vi "AutomatedBeamWatch.vi"   [LabVIEW 2019]
uses:
  C:/Program Files/Spiricon/BeamWatch/BeamWatch.Automation.dll
  Program Files/Spiricon/BeamWatch/BeamWatch.Automation.dll
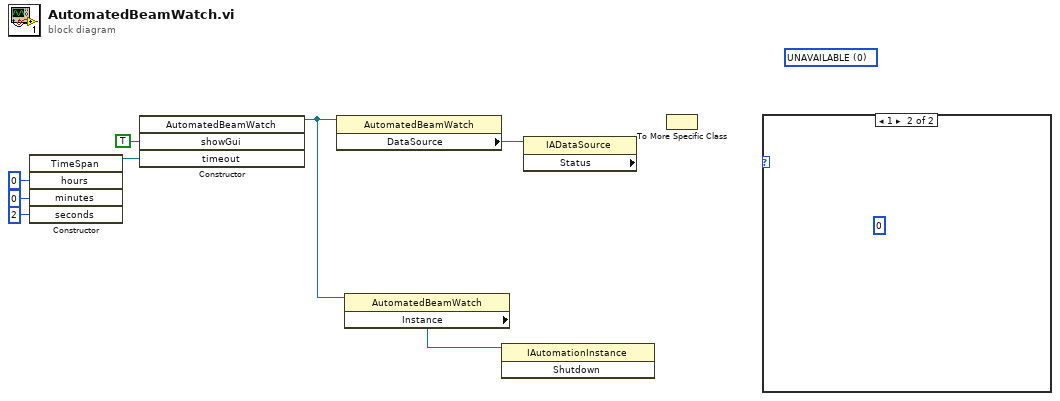
[diagram p0: block diagram]
diagram:
  (unwired) 0 items=["UNAVAILABLE", "RUNNING", "PAUSED"] ("Status")
  n1 = constructor class="TimeSpan"("hours"=0, "minutes"=0, "seconds"=2) -> (reference out=w4:refnum<k24>)  [unwired: 3 in, 5 out]
  n2 = constructor class="AutomatedBeamWatch"("showGui"=TRUE, "timeout"=w4) -> (reference out=w2:refnum<k24>)  [unwired: 3 in, 4 out]
  n3 = property class="AutomatedBeamWatch"(reference=w2) -> ("DataSource"=w3:refnum<k24>)  [unwired: 1 in, 2 out]
  n4 = property class="AutomatedBeamWatch"(reference=w2) -> ("Instance"=w1:refnum<k24>)  [unwired: 1 in, 2 out]
  n5 = invoke class="IAutomationInstance" method="Shutdown"(reference=w1) -> ()  [unwired: 2 in, 3 out]
  n6 = property class="IADataSource" props=["Status"](reference=w3) -> ()  [unwired: 1 in, 3 out]
  n7 = To More Specific Class() -> ()  [unwired: 3 in, 2 out]
  n8 = case shown="1" {
    selector: _ -> [_ _]
    frame 0, Default {
    }
    frame 1 {
      (unwired) 0
    }
  }
